vi "task_Keybut_detectAppCmd.vi"(8 "error in (no error)":errorcluster, 11 "Cmd Ref in":refnum<vi>[](array[refnum])) -> (0 "error IO":errorcluster, 3 "AppCmd":T1)   [LabVIEW 2015]
uses:
  UsrDefine/imt_app_cmd.ctl
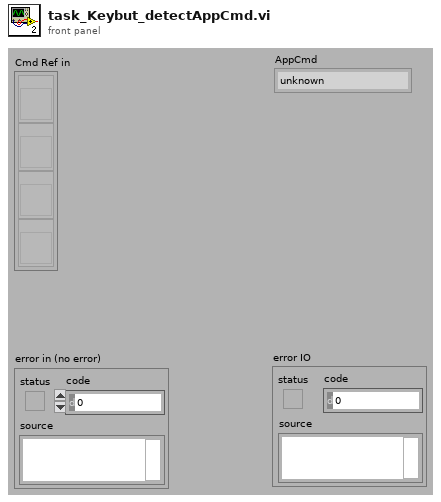
[diagram p1: front panel]
types:
  T1 = typedef "imt_app_cmd.ctl" = enum16{"unknown", "configHardware", "configDevice", "updateFirmware", "measurement"}
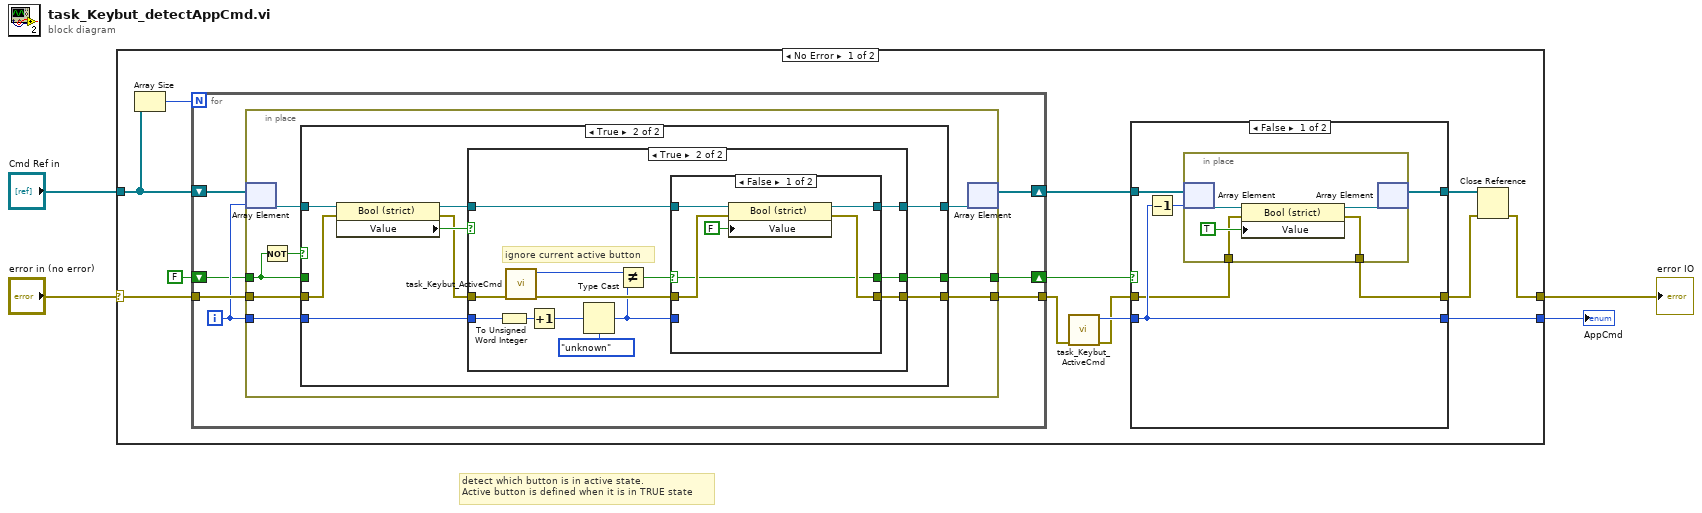
[diagram p0: block diagram]
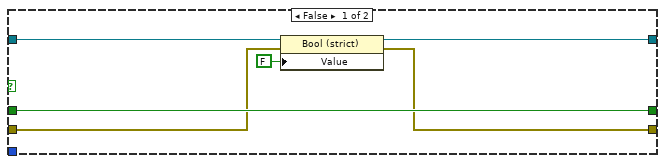
[diagram p3: hidden frame]
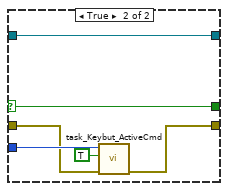
[diagram p5: hidden frame]
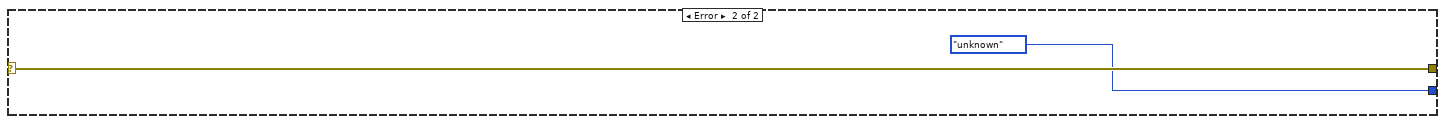
[diagram p6: hidden frame]
diagram:
  # "detect which button is in active state.\nActive button is defined when it is in TRUE state"
  n1 = case shown="No Error" "error in (no error)" {
    selector: "error in (no error)" -> [w17 w91]
    tunnel: "Cmd Ref in" -> [w15 _]
    tunnel: [w12 imt_app_cmd."unknown" ("AppCmd")] -> w2
    tunnel: [w9 w91] -> w1
    frame No Error {
      n2 = Array Size(array=w15) -> (size(s)=w16:i32)
      n3 = for {
        N: w16 -> [_]
        tunnel: w17 -> [w37]
        shift-right: [w35] -> w13
        shift-left: w15 -> [w38]
        tunnel: [w34] -> w6
        shift-right: [w33] -> w14
        shift-left: FALSE -> [w32]
        i -> [w36]
        n4 = in-place {
          in-place-border: w37 -> [w44]
          in-place-border: [w45] -> w34
          in-place-border: w36 -> [w43]
          in-place-border: [w41] -> w33
          in-place-border: w32 -> [w39]
          n5 = in-place-array #1(w38, w36) -> (w46:refnum<vi>)
          n6 = Not(x=w39) -> (.not. x?=w40:bool)
          n7 = case shown="True" w40 {
            tunnel: w46 -> [w51 w61]
            tunnel: [w48 w57] -> w45
            tunnel: w44 -> [w49 w56]
            tunnel: w43 -> [_ w55]
            tunnel: [w50 w54] -> w42
            tunnel: [w52 w53] -> w41
            tunnel: w39 -> [w52 _]
            frame False {
              n8 = property class="Bool (strict)"(reference=w51, error in=w49, "Value"=FALSE) -> (reference out=w50:refnum<vi>, error out=w48:errorcluster)
            }
            frame True {
              n9 = property class="Bool (strict)"(reference=w61, error in=w56) -> (reference out=w59:refnum<vi>, error out=w58:errorcluster, "Value"=w60:bool)
              n10 = case shown="True" w60 {
                selector: w60 -> [w62 _]
                tunnel: w59 -> [w64 w69]
                tunnel: w58 -> [w63 w73]
                tunnel: [w63 w67] -> w57
                tunnel: w55 -> [_ w72]
                tunnel: [w64 w68] -> w54
                tunnel: [w62 w66] -> w53
                frame False {
                }
                frame True {
                  # "ignore current active button"
                  n11 = To Unsigned Word Integer(number=w72) -> (unsigned 16bit integer=w77:u16)
                  n12 = call "task_Keybut_ActiveCmd.vi"("error in (no error)"=w73) -> ("error out"=w70:errorcluster, "AppCmd"=w76:T1)  [unwired: 9 in]
                  n13 = Increment(x=w77) -> (x+1=w75:u16)
                  n14 = Type Cast(type=imt_app_cmd."unknown" ("AppCmd"), x=w75) -> (*(type *) &x=w65:T1)
                  n15 = Not Equal?(x=w76, y=w65) -> (x != y?=w71:bool)
                  n16 = case shown="False" w71 {
                    selector: w71 -> [w78 w88]
                    tunnel: w70 -> [w82 w86]
                    tunnel: w69 -> [w83 w89]
                    tunnel: [w81 w89] -> w68
                    tunnel: [w80 w85] -> w67
                    tunnel: [w78 w88] -> w66
                    tunnel: w65 -> [_ w87]
                    frame False {
                      n17 = property class="Bool (strict)"(reference=w83, error in=w82, "Value"=FALSE) -> (reference out=w81:refnum<vi>, error out=w80:errorcluster)
                    }
                    frame True {
                      n18 = call "task_Keybut_ActiveCmd.vi"("error in (no error)"=w86, "update"=TRUE, "New AppCmd"=w87) -> ("error out"=w85:errorcluster)  [unwired: 7 in, 1 out]
                    }
                  }
                }
              }
            }
          }
          n19 = in-place-array #1(w42) -> (w35:refnum<vi>[])  [unwired: 1 out]
        }
      }
      n20 = call "task_Keybut_ActiveCmd.vi"("error in (no error)"=w6) -> ("error out"=w5:errorcluster, "AppCmd"=w7:T1)  [unwired: 9 in]
      n21 = case shown="False" w14 {
        tunnel: w13 -> [w23 w29]
        tunnel: w7 -> [w19 w31]
        tunnel: [w19 w31] -> w12
        tunnel: w5 -> [w18 w30]
        tunnel: [w22 w30] -> w10
        tunnel: [w21 w29] -> w11
        frame False {
          n22 = Decrement(x=w19) -> (x-1=w20:T1)
          n23 = in-place {
            in-place-border: w18 -> [w26]
            in-place-border: [w24] -> w22
            n24 = in-place-array #2(w23, w20) -> (w28:refnum<vi>)
            n25 = property class="Bool (strict)"(reference=w28, error in=w26, "Value"=TRUE) -> (reference out=w25:refnum<vi>, error out=w24:errorcluster)
            n26 = in-place-array #2(w25) -> (w21:refnum<vi>[])  [unwired: 1 out]
          }
        }
        frame True {
        }
      }
      n27 = Close Reference(reference=w11, error in (no error)=w10) -> (error out=w9:errorcluster)
    }
    frame Error {
    }
  }
  "AppCmd" <- w2
  "error IO" <- w1
